vi "SVPO Power Spectrum (N Ch DBL Array).vi"(0 "scaled signals [EU]":dbl[][](array[numeric]), 1 "sampling rate [Hz]":dbl=1.0, 2 "window":T7=1 items=["None"=0, "Hanning"=1, "Hamming"=2, "Blackman-Harris"=3, "Exact Blackman"=4, "Blackman"=5, "Flat Top"=6, "4 Term B-Harris "=7, "7 Term B-Harris"=8, "Low Sidelobe"=9, "Force"=64, "Exponential"=65, "Blackman Nuttall"=11, "Triangle"=30, "Bartlett-Hanning"=31, "Bohman"=32, "Parzen"=33, "Welch"=34, "Kaiser"=60, "Dolph-Chebyshev"=61, "Gaussian"=62], 9 "restart averaging? (F)":bool) -> (13 "averages completed":dbl, 14 "power spectra [EU^2 rms]":cluster{"f0":dbl, "df":dbl, "magnitude":dbl[]}[](array[cluster]) {"magnitude" format="%.2p"; "df" format="%.2p"; "f0" format="%.2p"}, 18 "spectrum info":T1={"channel name"="", "description"="", "x-axis units"=0, "spectral info"={"spectrum type"=enum."Power [Magnitude^2]", "linear/dB"=enum."linear", "window"=0, "window size"=0, "FFT size"=0}, "engineering units"=1, "custom label"="", "dB reference [EU]"=0.0, "peak units"=enum."rms", "weighting filter"=0, "spectral density?"=FALSE, "unit label"="", "spectrum skewed?"=FALSE, "complimentary spectrum units"=enum."none"} {"x-axis units" items=["Time (s)"=0, "Frequency-CB (Hz)"=1, "Frequency-CPB (Hz)"=1248, "Frequency-Arbitrary (Hz)"=2357, "Quefrency (s)"=2, "Revolutions (rev)"=3, "Order"=4, "Speed (RPM)"=11, "Speed (rad/s)"=21, "Index"=65535]; "weighting filter" items=["Linear", "A-weighting", "B-weighting", "C-weighting", "ITU-R 468-4", "Dolby", "CCITT", "C-message", "Wb", "Wc", "Wd", "We", "Wf", "Wh", "Wj", "Wk", "Wm", "AES17 20 kHz lowpass", "AES17 40 kHz lowpass", "AES17 20 kHz highpass", "AES17 40 kHz highpass"]; "dB reference [EU]" format="%.2f"; "engineering units" items=["custom..."=0, "V"=1, "A"=21, "C"=30, "pC"=31, "s"=32, "-"=29, "Pa"=2, "N"=20, "g"=3, "m/s^2"=4, "m/s"=5, "m"=6, "mm/s"=12, "mm"=13, "micron/s"=14, "micron"=15, "in/s^2"=7, "in/s"=8, "in"=9, "mil/s"=10, "mil"=11, "rad/s^2"=16, "rad/s"=17, "rad"=18, "deg/s^2"=26, "deg/s"=27, "deg"=28, "RPM"=22, "cycle/s^2"=23, "Hz"=24, "cycle"=25, "strain"=19]; "spectral info"."window" items=["None "=0, "Hanning"=1, "Hamming"=2, "Blackman-Harris"=3, "Exact Blackman"=4, "Blackman"=5, "Flat Top"=6, "4 Term B-Harris "=7, "7 Term B-Harris"=8, "Low Sidelobe"=9, "Force - Exponential"=10, "Gaussian"=62]})   [LabVIEW 2017]
doc: "Computes the linear RMS-averaged power spectrum of <B>scaled signal [EU]</B> in a linear scale. Use the power spectrum to quantify signal components as a function of frequency. Use this VI on embedded targets that have limited computational resources. Wire data to the <B>scaled signal [EU]</B> input to determine the polymorphic instance to use or manually select the instance."
uses:
  <vilib>/addons/_NISVFA/_Shared subVIs/Controls/svc_Window.ctl
  <vilib>/addons/_NISVFA/_Shared subVIs/Controls/svc_Spectrum Info.ctl
  <vilib>/addons/_NISVFA/_Shared subVIs/Controls/svc_X-Axis Units.ctl
  <vilib>/addons/_NISVFA/_Shared subVIs/Controls/svc_Spectrum Type.ctl
  <vilib>/addons/_NISVFA/_Shared subVIs/Controls/svc_Engineering Units Text Ring.ctl
  <vilib>/addons/_NISVFA/_Shared subVIs/Controls/svc_Weighting Filter Text Ring.ctl
  <vilib>/addons/_NISVFA/_Shared subVIs/Controls/svc_Complimentary Spectrum Units.ctl
  <vilib>/Analysis/2dsp.llb/Power Spectrum (DBL).vi
  <vilib>/Analysis/4window.llb/Force Window.vi
  <vilib>/Analysis/4window.llb/Force Window (DBL).vi
  <vilib>/Analysis/4window.llb/Exponential Window.vi
  <vilib>/Analysis/4window.llb/Exponential Window (DBL).vi
  <vilib>/Utility/error.llb/Error Cluster From Error Code.vi
  <vilib>/Analysis/0measdsp.llb/Scaled Time Domain Window.vi
  <vilib>/Analysis/0measdsp.llb/Scaled Time Domain Window (DBL).vi
  <vilib>/addons/_NISVFA/_Spectrum Processing/subVIs/svfa_Spectrum Info Window to windowTd Type Def.vi
  <vilib>/Analysis/NI_AALPro.lvlib
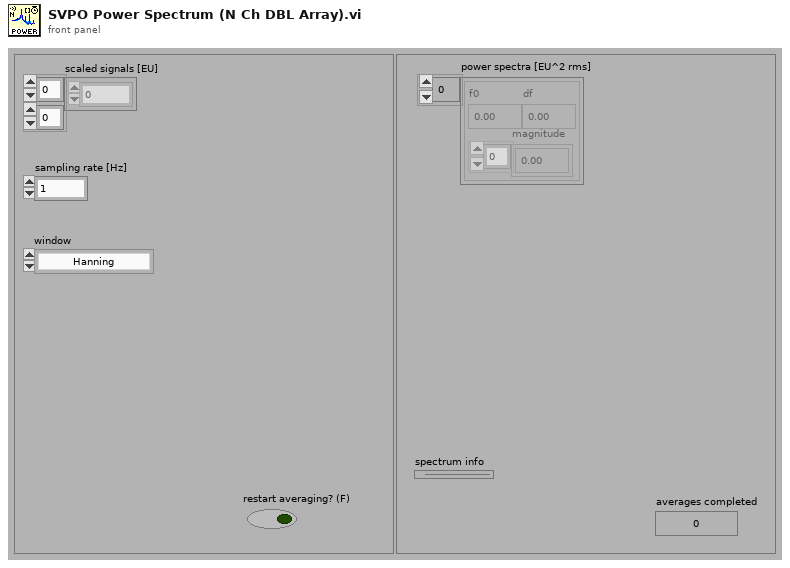
[diagram p1: front panel]
types:
  T1 = typedef "svc_Spectrum Info.ctl" = cluster{"channel name":string, "description":string, "x-axis units":T2, "spectral info":cluster{"spectrum type":T3, "linear/dB":enum16{"linear", "dB"}, "window":u16, "window size":i32, "FFT size":i32}, "engineering units":T4, "custom label":string, "dB reference [EU]":dbl, "peak units":enum16{"rms", "peak", "peak-peak"}, "weighting filter":T5, "spectral density?":bool, "unit label":string, "spectrum skewed?":bool, "complimentary spectrum units":T6}
  T2 = typedef "svc_X-Axis Units.ctl" = u16
  T3 = typedef "svc_Spectrum Type.ctl" = enum16{"FFT Spectrum [complex]", "Amplitude [Magnitude]", "Power [Magnitude^2]", "Cross Spectrum [complex]", "Frequency Response [Complex]"}
  T4 = typedef "svc_Engineering Units Text Ring.ctl" = u16
  T5 = typedef "svc_Weighting Filter Text Ring.ctl" = u16
  T6 = typedef "svc_Complimentary Spectrum Units.ctl" = enum16{"none", "radians", "degrees", "cycles", "imaginary"}
  T7 = typedef "svc_Window.ctl" = u32
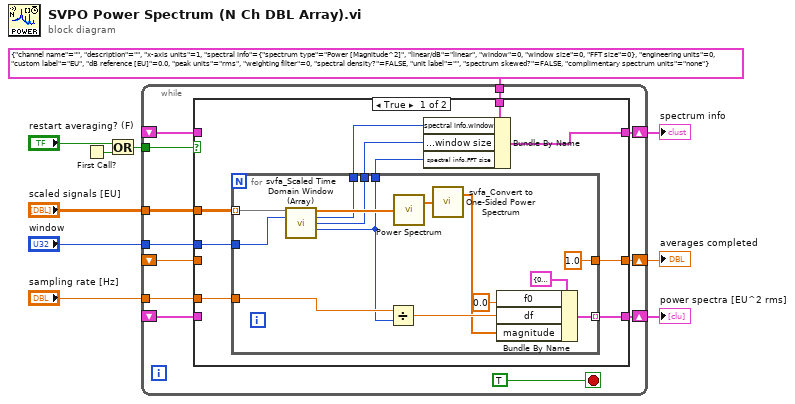
[diagram p0: block diagram]
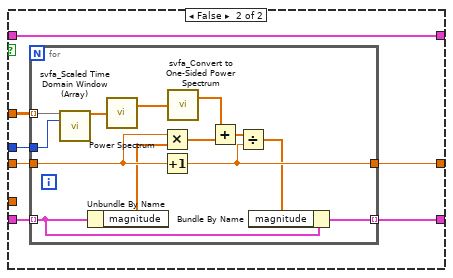
[diagram p2: hidden frame]
diagram:
  n1 = First Call?() -> (First Call?: T/F=w5:bool)
  n2 = Or(x="restart averaging? (F)", y=w5) -> (x .or. y?=w4:bool)
  n3 = while {
    tunnel: "window" -> [w21]
    shift-right: [w13] -> w2
    shift-left: _ -> [w11]
    tunnel: w4 -> [w14]
    tunnel: "sampling rate [Hz]" -> [w19]
    tunnel: "scaled signals [EU]" -> [w18]
    shift-right: [w20] -> w9
    shift-left: _ -> [w16]
    shift-right: [w17] -> w1
    shift-left: _ -> [w15]
    tunnel: T1 {"channel name"="", "description"="", "x-axis units"=1, "spectral info"={"spectrum type"=enum."Power [Magnitude^2]", "linear/dB"=enum."linear", "window"=0, "window size"=0, "FFT size"=0}, "engineering units"=0, "custom label"="EU", "dB reference [EU]"=0.0, "peak units"=enum."rms", "weighting filter"=0, "spectral density?"=FALSE, "unit label"="", "spectrum skewed?"=FALSE, "complimentary spectrum units"=enum."none"} ("spectrum info in") -> [w12]
    stop <- TRUE stop-if-true
    n4 = case shown="True" w14 {
      tunnel: w18 -> [w32 w53]
      tunnel: w21 -> [w24 w52]
      tunnel: [w31 w47] -> w20
      tunnel: w19 -> [w30 _]
      tunnel: [w29 w48] -> w17
      tunnel: w16 -> [_ w51]
      tunnel: w15 -> [_ w50]
      tunnel: [w28 w49] -> w13
      tunnel: w12 -> [w27 _]
      tunnel: w11 -> [_ w49]
      frame True {
        n5 = for {
          tunnel: w32 -> [w41] mode=indexing
          tunnel: [w44] -> w31 mode=indexing
          tunnel: w24 -> [w40]
          tunnel: w30 -> [w43]
          tunnel: [1.0 ("averages completed out")] -> w29
          tunnel: [w35] -> w26
          tunnel: [w34] -> w25
          tunnel: [w33] -> w23
          n6 = call <vilib>:"svfa_Scaled Time Domain Window (Array).vi"("input signal"=w41, "window"=w40) -> ("windowed signal"=w39:dbl[], "dup window"=w33:T7, "window length"=w34:i32, "FFT length"=w35:i32)  [unwired: 8 in, 2 out]
          n7 = Divide(x=w43, y=w35) -> (x/y=w42:dbl)
          n8 = call-poly <vilib>:"Power Spectrum.vi"("X"=w39) -> ("Power Spectrum"=w45:dbl[])  [unwired: 1 out]
          n9 = call <vilib>:"svfa_Convert to One-Sided Power Spectrum.vi"("two-sided power spectrum"=w45) -> ("one-sided power spectrum"=w38:dbl[])  [unwired: 1 out]
          n10 = Bundle By Name(cluster=cluster{"f0":dbl, "df":dbl, "magnitude":dbl[]} {"f0"=0.0, "df"=0.0, "magnitude"=[]} ("power spectrum [dB EU]"), "f0"=0.0, "df"=w42, "magnitude"=w38) -> (w44:cluster{"f0":dbl, "df":dbl, "magnitude":dbl[]})
        }
        n11 = Bundle By Name(cluster=w27, "spectral info.window"=w23, "spectral info.window size"=w25, "spectral info.FFT size"=w26) -> (w28:T1)
      }
      frame False {
        n12 = for {
          tunnel: w53 -> [w65] mode=indexing
          tunnel: w52 -> [w64]
          tunnel: w51 -> [w57] mode=indexing
          tunnel: w50 -> [w59]
          tunnel: [w58] -> w48
          tunnel: [w54] -> w47 mode=indexing
          n13 = call <vilib>:"svfa_Scaled Time Domain Window (Array).vi"("input signal"=w65, "window"=w64) -> ("windowed signal"=w63:dbl[])  [unwired: 8 in, 5 out]
          n14 = Unbundle By Name(w57) -> ("magnitude"=w56:dbl[])
          n15 = call-poly <vilib>:"Power Spectrum.vi"("X"=w63) -> ("Power Spectrum"=w66:dbl[])  [unwired: 1 out]
          n16 = Multiply(x=w59, y=w56) -> (x*y=w62:dbl[])
          n17 = Increment(x=w59) -> (x+1=w58:dbl)
          n18 = call <vilib>:"svfa_Convert to One-Sided Power Spectrum.vi"("two-sided power spectrum"=w66) -> ("one-sided power spectrum"=w60:dbl[])  [unwired: 1 out]
          n19 = Add(x=w60, y=w62) -> (x+y=w61:dbl[])
          n20 = Divide(x=w61, y=w58) -> (x/y=w55:dbl[])
          n21 = Bundle By Name(cluster=w57, "magnitude"=w55) -> (w54:cluster{"f0":dbl, "df":dbl, "magnitude":dbl[]})
        }
      }
    }
  }
  "power spectra [EU^2 rms]" <- w9
  "averages completed" <- w1
  "spectrum info" <- w2
